vi "Ctor.vi"(8 "error in (no error)":errorcluster, 10 "Port (8085)":u16=8085, 11 "Host (localhost)":string="127.0.0.1") -> (0 "error out":errorcluster, 3 "OpenHW out":refnum<class "OpenHW.lvclass">)   [LabVIEW 2022 SP3, in "open-hw-mon-lv.lvlib" / "OpenHW.lvclass"]
uses:
  OpenHW.lvclass
  OpenHW.lvclass/OpenHW.ctl
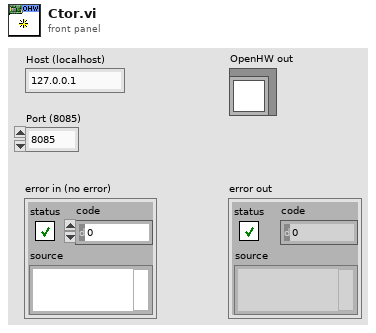
[diagram p1: front panel]
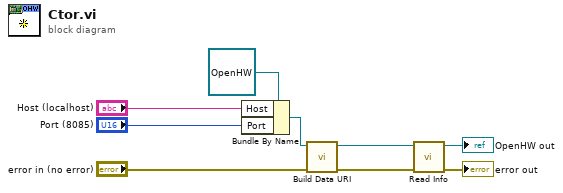
[diagram p0: block diagram]
diagram:
  n1 = Bundle By Name(cluster=refnum<class "OpenHW.lvclass"> refnum ("OpenHW in"), "Host"="Host (localhost)", "Port"="Port (8085)") -> (w6:refnum<class "OpenHW.lvclass">)
  n2 = call "Build Data URI.vi"("error in (no error)"="error in (no error)", "OpenHW in"=w6) -> ("error out"=w3:errorcluster, "OpenHW out"=w4:refnum<class "OpenHW.lvclass">)  [unwired: 8 in]
  n3 = call "Read Info.vi"("error in (no error)"=w3, "OpenHW in"=w4) -> ("error out"=→"error out":errorcluster, "OpenHW out"=→"OpenHW out":refnum<class "OpenHW.lvclass">)  [unwired: 8 in]
